vi "Experiment_Disp_ AttTrav.vi"() -> ()   [LabVIEW 2009]
uses:
  <vilib>/imath/engines/lvmath2/RunTimeEngine/ErrorHandling/NIMS_Finalize Error.vi
  <vilib>/imath/engines/lvmath2/RunTimeEngine/Parser/MC_Version.vi
  <vilib>/imath/engines/lvmath/Functions/Error Handling/error.ctl
  <vilib>/imath/engines/lvmath2/RunTimeEngine/RangeToken/NIMS_Range.vi
  <instcachedir>/0/NIMS_Range_6D647EC16A744C98B5DE1D649A2D648D.lvgen/NIMS_Range_6D647EC16A744C98B5DE1D649A2D648D_001.vi
  <vilib>/imath/engines/lvmath/Functions/Error Handling/MergeErrorsWrapper.vi
  <vilib>/imath/engines/lvmath2/RunTimeEngine/VariableToken/NIMS_VariableToken_CondDefined.vi
  <instcachedir>/0/NIMS_VariableToken_CondDefined_5641E79000FB4D628475532441475385.lvgen/NIMS_VariableToken_CondDefined_5641E79000FB4D628475532441475385_002.vi
  <instcachedir>/0/NIMS_VariableToken_CondDefined_5641E79000FB4D628475532441475385.lvgen/NIMS_VariableToken_CondDefined_5641E79000FB4D628475532441475385_001.vi
  <vilib>/imath/engines/lvmath/Functions/Error Handling/MC_Mask_Errors.vi
  <vilib>/imathl/engines/lvmath/Functions/Error Handling/Create Error.vi
  <vilib>/imath/engines/lvmath2/RunTimeEngine/ReplaceToken/NIMS_Replace - V(S)=S.vi
  <instcachedir>/0/NIMS_Replace - V(S)=S_670A9E0533664C1D848C8E58B3321B6A.lvgen/NIMS_Replace - V(S)=S_670A9E0533664C1D848C8E58B3321B6A_000.vi
  <vilib>/imath/engines/lvmath2/RunTimeEngine/ReplaceToken/NIMS_Replace - Size Check _(_)=S.vi
  <instcachedir>/0/NIMS_Replace - Size Check _(_)=S_8596181D73404097BAB9CBB006194BB0.lvgen/NIMS_Replace - Size Check _(_)=S_8596181D73404097BAB9CBB006194BB0_001.vi
  <vilib>/imath/engines/lvmath2/RunTimeEngine/ReplaceToken/NIMS_Replace - Check Linear.vi
  <instcachedir>/0/NIMS_Replace - Check Linear_9243CBB174894FF6977027453DA6955E.lvgen/NIMS_Replace - Check Linear_9243CBB174894FF6977027453DA6955E_001.vi
  <vilib>/imath/engines/lvmath2/RunTimeEngine/VariableToken/NIMS_VariableToken_CondDefinedDefinedByReplace.vi
  <instcachedir>/0/NIMS_VariableToken_CondDefinedDefinedByReplace_D162CFFC24174562A9FEA619A91E1A56.lvgen/NIMS_VariableToken_CondDefinedDefinedByReplace_D162CFFC24174562A9FEA619A91E1A56_001.vi
  <instcachedir>/0/NIMS_Replace - V(S)=S_670A9E0533664C1D848C8E58B3321B6A.lvgen/NIMS_Replace - V(S)=S_670A9E0533664C1D848C8E58B3321B6A_001.vi
  <instcachedir>/0/NIMS_Replace - Size Check _(_)=S_8596181D73404097BAB9CBB006194BB0.lvgen/NIMS_Replace - Size Check _(_)=S_8596181D73404097BAB9CBB006194BB0_002.vi
  <instcachedir>/0/NIMS_Replace - Check Linear_9243CBB174894FF6977027453DA6955E.lvgen/NIMS_Replace - Check Linear_9243CBB174894FF6977027453DA6955E_002.vi
  <instcachedir>/0/NIMS_VariableToken_CondDefinedDefinedByReplace_D162CFFC24174562A9FEA619A91E1A56.lvgen/NIMS_VariableToken_CondDefinedDefinedByReplace_D162CFFC24174562A9FEA619A91E1A56_002.vi
  <vilib>/imath/engines/lvmath2/RunTimeEngine/CommandStatement/MC_CommandStatement_break.vi
  <vilib>/imath/engines/lvmath2/RunTimeEngine/Managers/WorkSpace/UID Generator.vi
  <vilib>/imath/engines/lvmath2/RunTimeEngine/Managers/SymbolTable/Clear UID.vi
  <instcachedir>/0/NIMS_VariableToken_CondDefined_5641E79000FB4D628475532441475385.lvgen/NIMS_VariableToken_CondDefined_5641E79000FB4D628475532441475385_003.vi
  <instcachedir>/0/NIMS_Replace - V(S)=S_670A9E0533664C1D848C8E58B3321B6A.lvgen/NIMS_Replace - V(S)=S_670A9E0533664C1D848C8E58B3321B6A_002.vi
  <instcachedir>/0/NIMS_Replace - Size Check _(_)=S_8596181D73404097BAB9CBB006194BB0.lvgen/NIMS_Replace - Size Check _(_)=S_8596181D73404097BAB9CBB006194BB0_003.vi
  <vilib>/imath/engines/lvmath2/RunTimeEngine/ArithmeticOperatorToken/NIMS_ArithmeticOperator_power(S).vi
  <instcachedir>/0/NIMS_ArithmeticOperator_power(S)_A502679C095F4520BDC53E297C98A9BD.lvgen/NIMS_ArithmeticOperator_power(S)_A502679C095F4520BDC53E297C98A9BD_000.vi
  <instcachedir>/0/NIMS_Replace - Check Linear_9243CBB174894FF6977027453DA6955E.lvgen/NIMS_Replace - Check Linear_9243CBB174894FF6977027453DA6955E_003.vi
  <instcachedir>/0/NIMS_VariableToken_CondDefinedDefinedByReplace_D162CFFC24174562A9FEA619A91E1A56.lvgen/NIMS_VariableToken_CondDefinedDefinedByReplace_D162CFFC24174562A9FEA619A91E1A56_003.vi
  <vilib>/imath/engines/lvmath2/RunTimeEngine/LocalVariableDefStatement/MC_LocalVariableDefStatement_Display.vi
  <vilib>/imath/engines/lvmath2/RunTimeEngine/RunTimeType/NIMS_RunTimeType_From StrictType (excl LVString).vi
  <vilib>/imath/engines/lvmath2/RunTimeEngine/VariableToken/Read/NIMS_Get Elements - RV(_) - Check.vi
  <instcachedir>/0/NIMS_Get Elements - RV(_) - Check_60F12861D0564803969A5D0D0D1716CD.lvgen/NIMS_Get Elements - RV(_) - Check_60F12861D0564803969A5D0D0D1716CD_002.vi
  <vilib>/imath/engines/lvmath2/RunTimeEngine/Managers/SymbolTable/NIMS_WorkSpace.lvlib
panel:
  out "error out":errorcluster
  out "error out":errorcluster
  out "error out":errorcluster
  in  "?":enum32{"TRANSMISSION LINE DEMONSTRATOR"}(tab)
  out "?":cluster{"Y":dbl[], "Y":dbl[]}[](graph)
  in  "Delay Time (s)":dbl min=0.0 step=0.005
  in  "HELP FOR TLD":bool
  in  "?":enum32{"OSCILOSCOPE"}(tab)
  out "?":cluster{"Y":dbl[], "Y":dbl[]}[](graph)
  in  "HELP FOR CRO":bool
  in  "?":enum32{"SOURCE"}(tab)
  out "?":cluster{"Y":dbl[], "Y":dbl[]}[](graph)
  in  "HELP FOR SOURCE":bool
  in  "?":bool
  # "Transmission line demonstrator"
  # "Osciloscope"
  # "Function generator"
  # "ON"
  # "OFF"
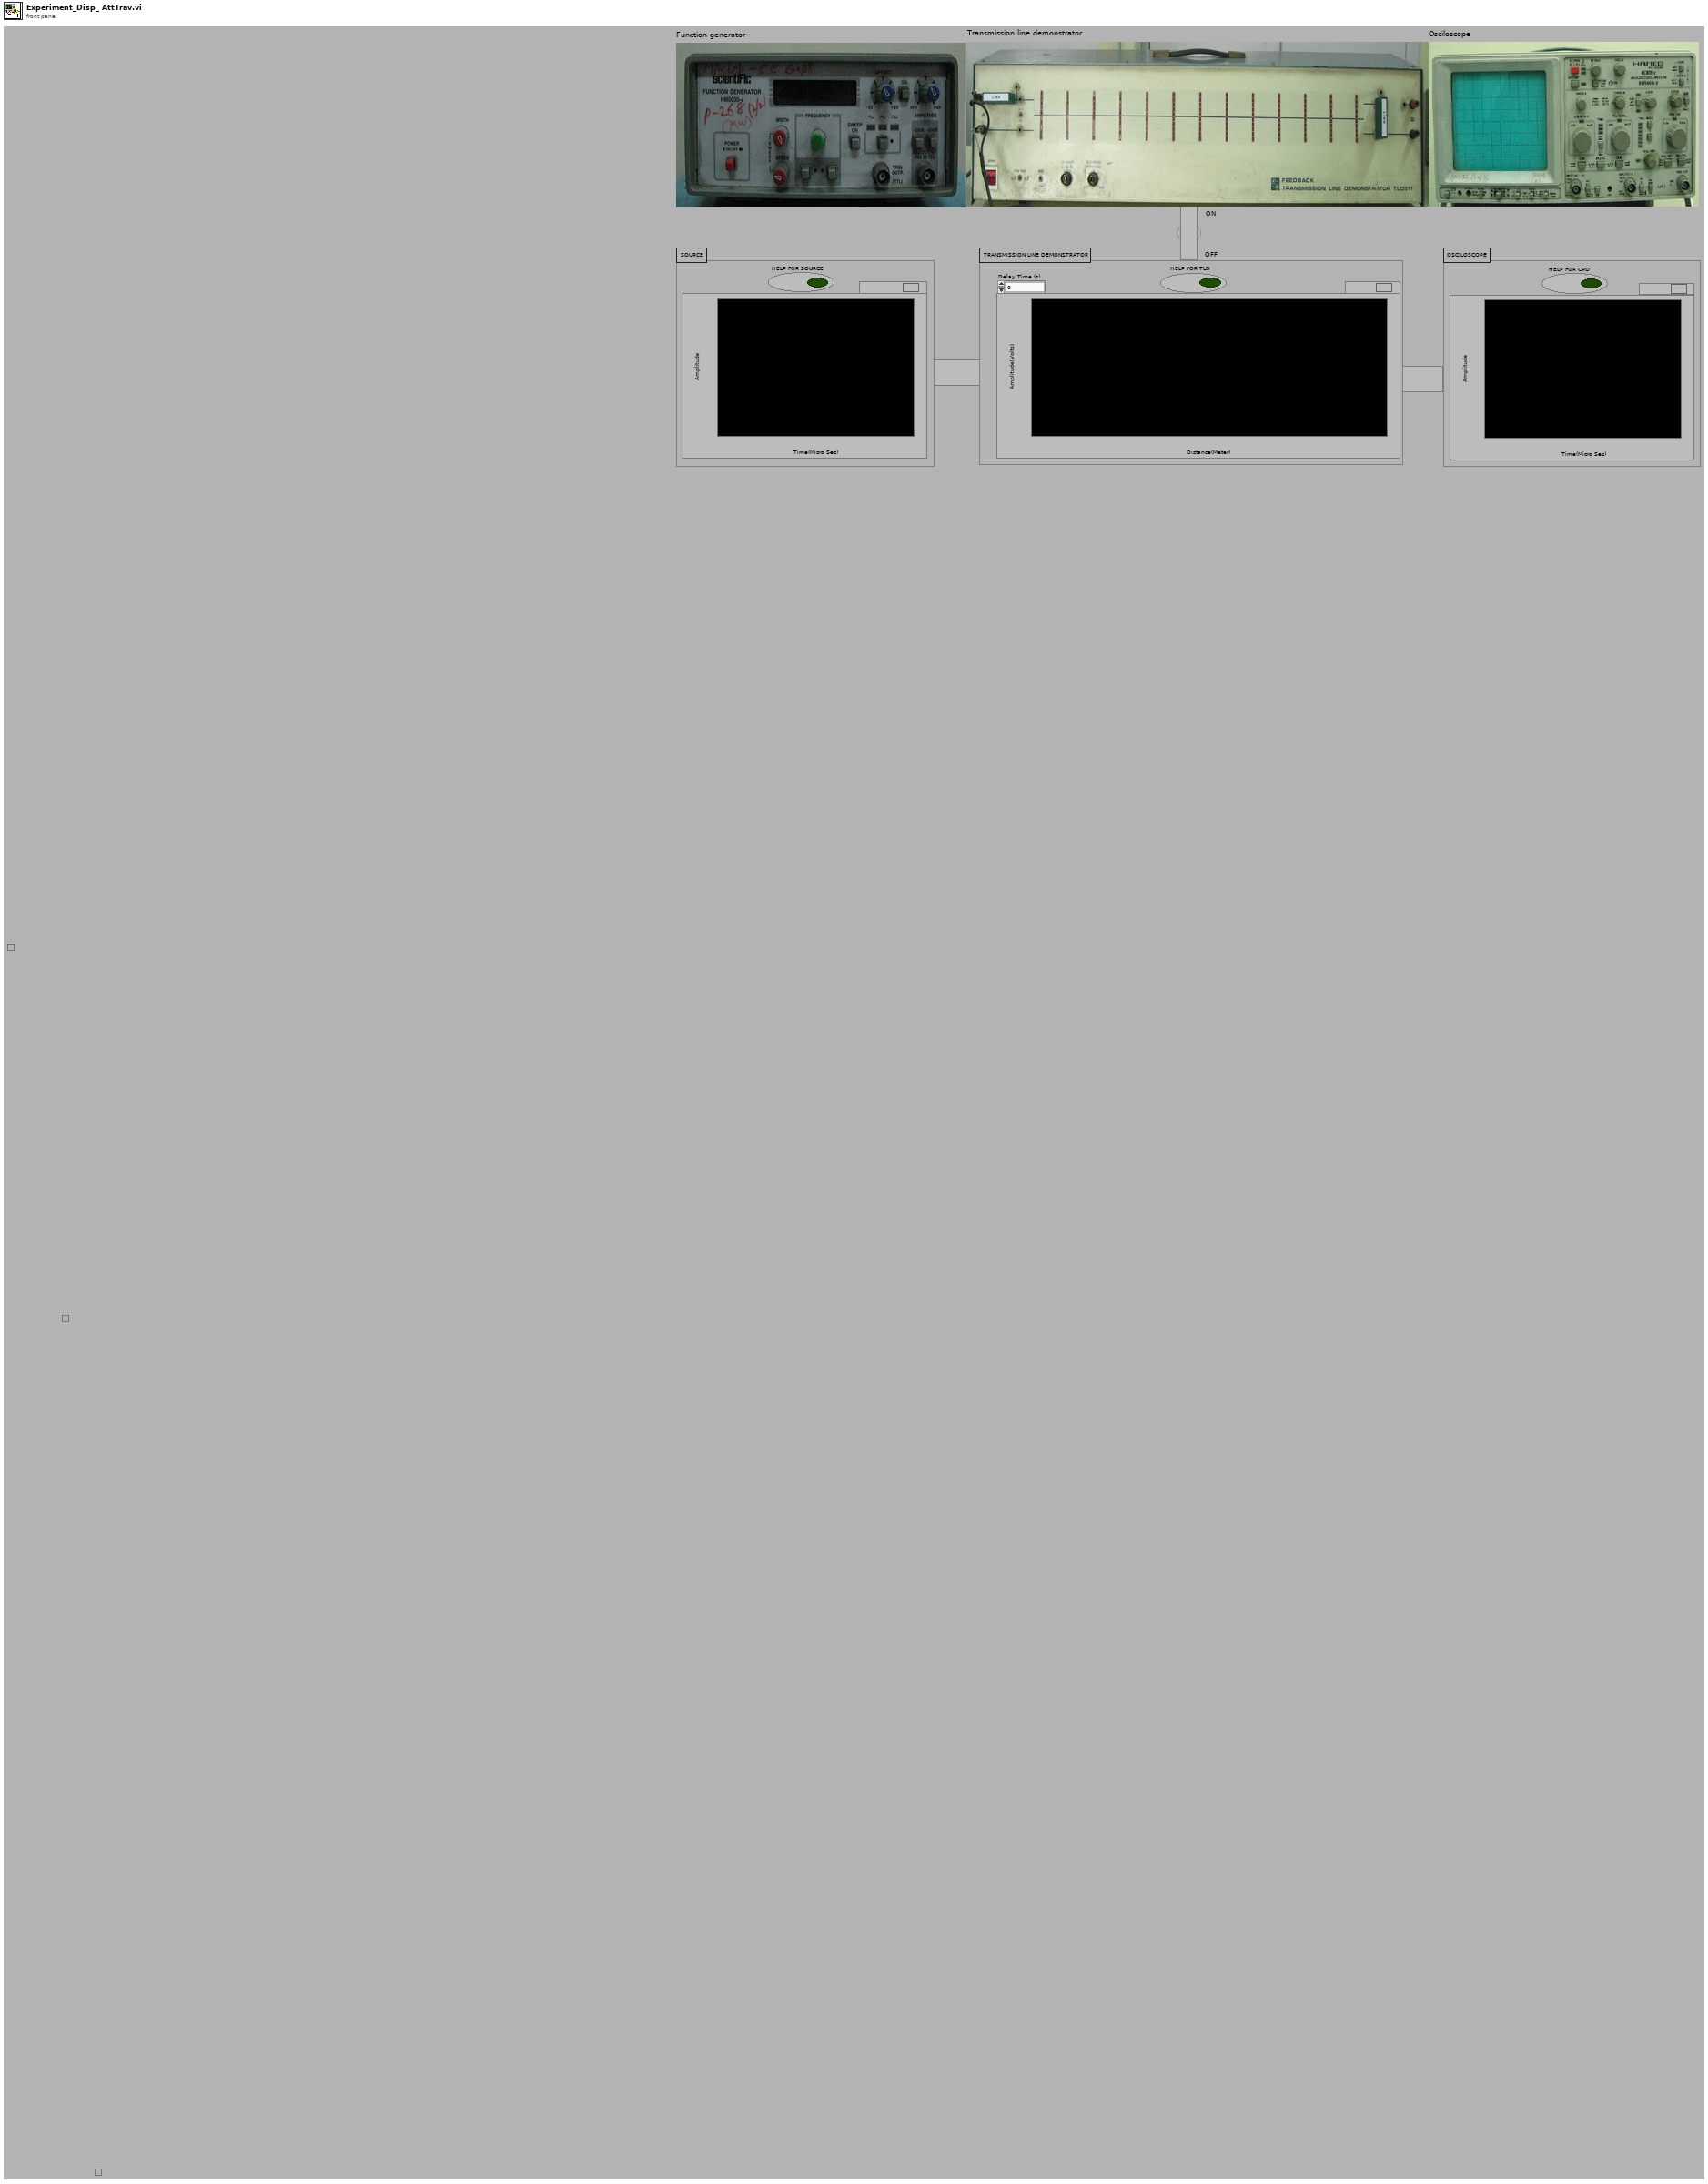
[diagram p1: front panel]
types:
  T1 = typedef "error.ctl" = enum16{"No Error", "Problem", "Unused002", "Incorrect number of parameters", "Function not defined for non-numeric types", "Unused005", "Function only defined for character arrays", "Function not defined for boolean, character, or single precision", "Function not defined for complex types", "Not a valid operation", "Inputs must be scalar", "Input matrices are not the same size", "Unused012", "Input matrices must be nonnegative integers of the same type", "Arguments must be non-negative integers less than bitmax", "Number to complement must be less than 2^N", "Bit to get is outside range", "Bit to set is outside range", "Input must be real type ", "At least one parameter must be scalar", "Unused020", "Function not defined for\nhigher dimensional matrices.", "Invalid attributes", "Wrong Type of Input Arguments", "Wrong Argument Option", "Unused025", "Indices must be real positive integers", "Unused027", "Number of elements must be the same for indices and values", "Unused029", "Cannot resize a 2D matrix with a linear index", "Unknown variable or symbol", "Indices out of range", "Empty matrix deletion can not be used with two indices", "Number of rows and columns must be the same for indices and values.", "Complex cannot be converted to Boolean", "Char cannot be converted to Boolean", "int64 cannot be converted to Boolean", "uint64 cannot be converted to Boolean", "Unused039", "Unused040", "All rows must have the same number of columns", "Incompatible types", "Invalid matrix dimensions", "Dimension must be 1 or 2", "Base must be an integer between 2 and 36", "Invalid input", "Square matrix required", "Function 'timerstart' must be called before 'timerstop'", "Arguments must be positive real", "Step must not be zero", "Wrong number of input arguments", "Wrong number of output arguments", "Unused053", "Input scalar must be >= 0", "Input scalar must be positive", "Input scalar must not be 0", "Input scalar must be in range [0,1]", "Unused058", "Input must be a vector", "Unused060", "Empty vector error", "All elements must be in domain [-1,1]", "All real elements of input vector must be >= 0", "All elements of input vector must be positive", "Values of input vectors are not compatible", "Unused066", "Input vector must be an increasing vector", "Unused068", "Unused069", "Lenths of two input vectors are not compatible", "Unused071", "Empty matrix error", "Unused073", "Unused074", "Unused075", "Unused076", "Unused077", "Size of input matrix is incompatible with input size", "Invalid format specifier", "Unused080", "Unused081", "Unused082", "Unused083", "Unused084", "Unused085", "RunTime: MathScript could not be compiled", "Unknown function", "Only scalars and strings supported", "Unused089", "Unused090", "Range is too large", "End used without variable", "Function not available (RTE)", "Custom user error", "Arguments must be integers less than bitmax", "Shared library not found", "Header file not found", "Shared library already loaded", "Shared library not loaded", "Shared library function not found", "Shared library string return problem", "Problem calling shared library function", "Problem loading shared library from OS", "Problem parsing shared library header file", "Shared library incompatible types", "Shared library unsupported return type", "Shared library function not exported", "Shared library unsupported input type", "Problem unloading shared library from OS", "Function only available from UI", "Invalid function specified in argument", "An internal error has occurred", "Invalid object", "Invalid property", "Read-only property", "A break command has occurred", "A continue command has occurred", "A return command has occurred", "ode: times parameter invalid", "Unused120", "Function not found in file", "Reserved keyword cannot be defined as variable", "Reserved keyword cannot be defined as a function or script", "Arguments must be string literals", "Function not supported on this platform", "All columns must have the same number of rows", "Function ignored in RTE warning", "Cannot use : as a parameter that is not a variable", "Output can't be coerced to requested type", "Function not supported on current target", "Variable dependent on an unwired function input", "Unused132", "Unused133", "Unused134", "Unused135", "Unused136", "Unused137", "Unused138", "Unused139", "Unused140", "Unused141", "Unused142", "Unused143", "Unused144", "Unused145", "Unused146", "MathScript parser DLL missing", "MathScript requires LabVIEW Full", "MathScript license is invalid or missing"}
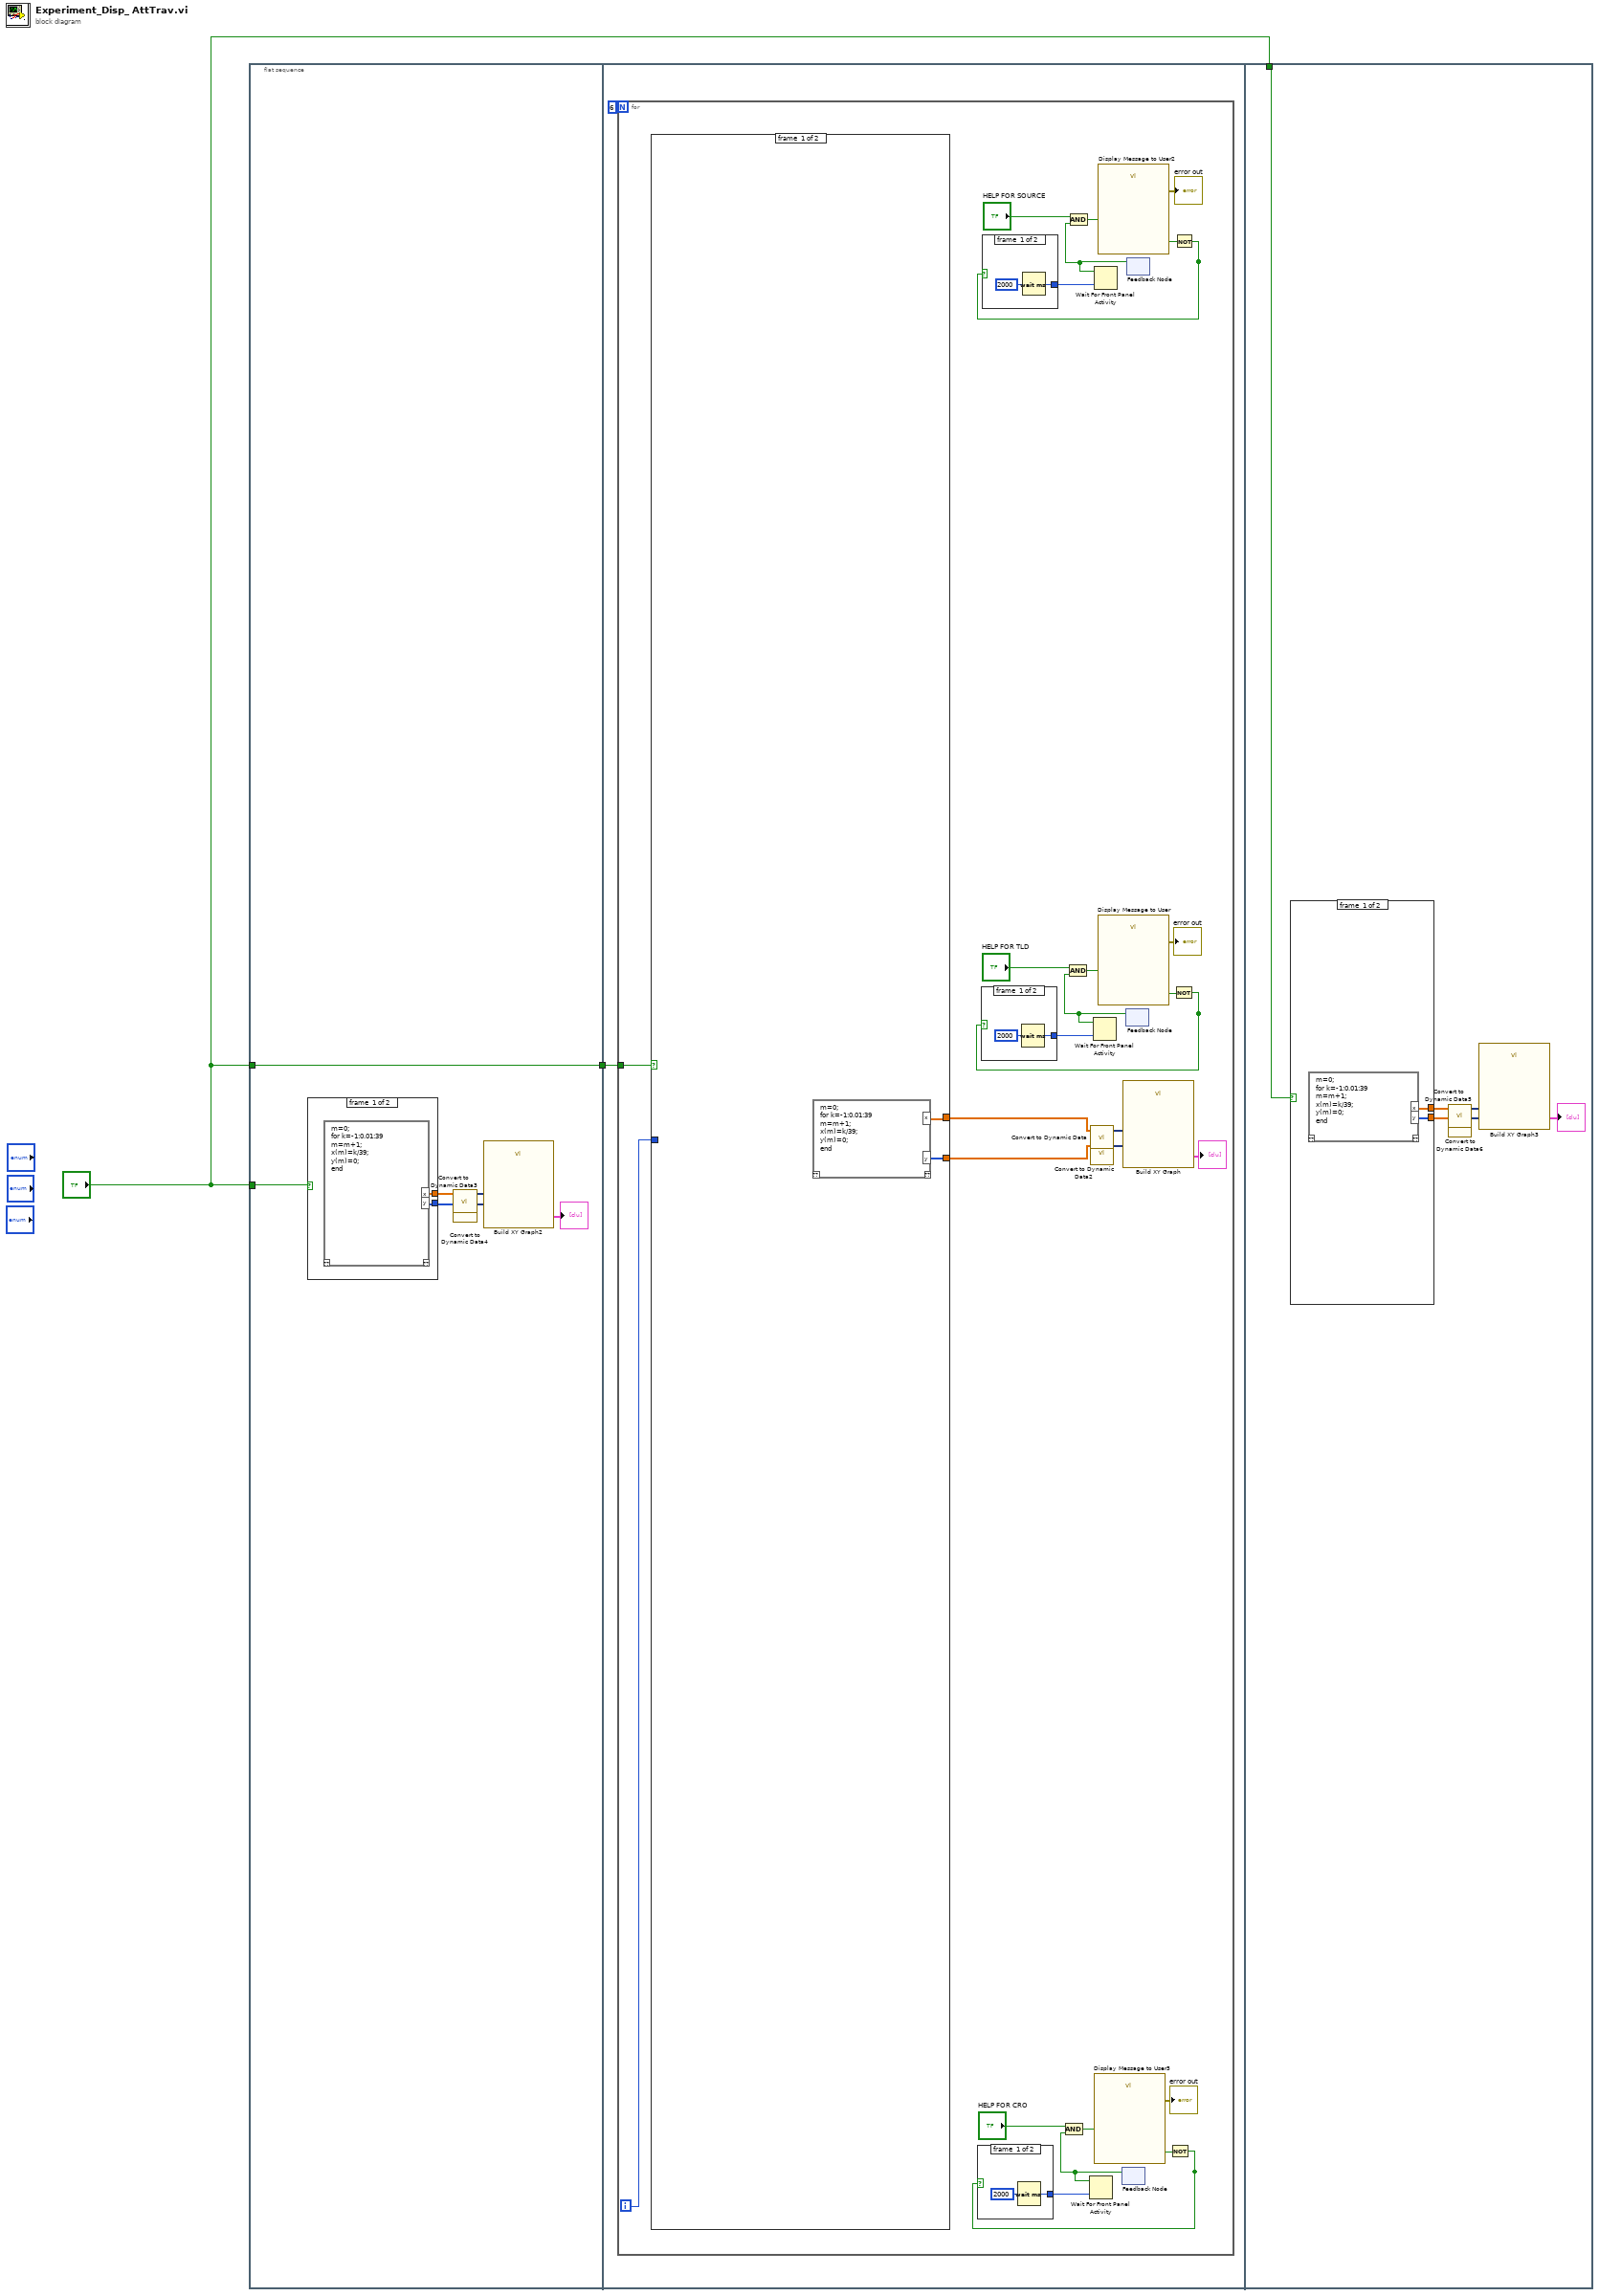
[diagram p0: block diagram]
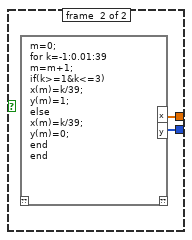
[diagram p2: hidden frame]
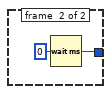
[diagram p3: hidden frame]
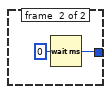
[diagram p4: hidden frame]
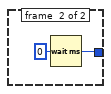
[diagram p5: hidden frame]
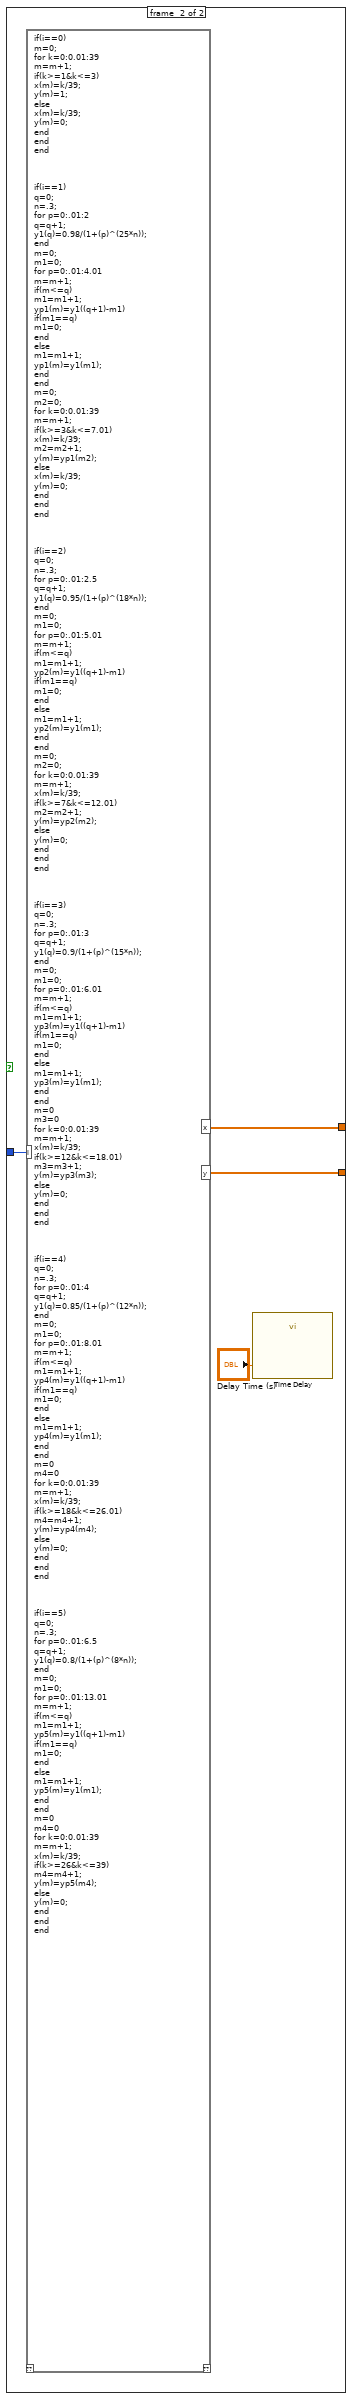
[diagram p6: hidden frame]
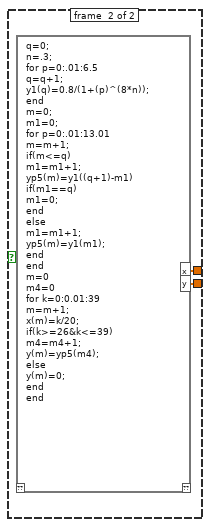
[diagram p7: hidden frame]
diagram:
  n1 = flat-sequence {
    tunnel: [w4] -> w2
    tunnel: "?" -> [w4]
    tunnel: "?" -> [w3]
    tunnel: w2 -> [w338]
    tunnel: "?" -> [w3370]
    frame #0 {
      n2 = case shown="True" w3 {
        tunnel: [w10 w146] -> w9
        tunnel: [w11 w145] -> w7
        frame #0 {
          n3 = mathscript code="m=0;\nfor k=-1:0.01:39\nm=m+1;\nx(m)=k/39;\ny(m)=0;\nend"() -> ("x"=w10:dbl[], "y"=w11:i32[])  [unwired: 1 in, 1 out]
        }
        frame #1 {
          n4 = mathscript code="m=0;\nfor k=-1:0.01:39\nm=m+1;\nif(k>=1&k<=3)\nx(m)=k/39;\ny(m)=1;\nelse\nx(m)=k/39;\ny(m)=0;\nend\nend"() -> ("x"=w146:dbl[], "y"=w145:i32[])  [unwired: 1 in, 1 out]
        }
      }
      n5 = call "Convert to Dynamic Data3"("Array"=w9) -> ("Dynamic Data Type"=w8:dynamicdata)  [unwired: 3 in]
      n6 = call "Convert to Dynamic Data4"("Array"=w7) -> ("Dynamic Data Type"=w6:dynamicdata)  [unwired: 3 in]
      n7 = call "Build XY Graph2"("Y Input"=w6, "X Input"=w8) -> ("XY Graph"=→"?":cluster{"Y":dbl[], "Y":dbl[]}[])  [unwired: 8 in, 1 out]
    }
    frame #1 {
      n8 = for {
        N: 6 -> [_]
        tunnel: w338 -> [w361]
        i -> [w367]
        n9 = case shown="True" w361 {
          tunnel: w367 -> [_ w518]
          tunnel: [w381 w517] -> w363
          tunnel: [w380 w516] -> w362
          frame #0 {
            n10 = mathscript code="m=0;\nfor k=-1:0.01:39\nm=m+1;\nx(m)=k/39;\ny(m)=0;\nend"() -> ("x"=w381:dbl[], "y"=w380:i32[])  [unwired: 1 in, 1 out]
          }
          frame #1 {
            n11 = mathscript code="if(i==0)\nm=0;\nfor k=0:0.01:39\nm=m+1;\nif(k>=1&k<=3)\nx(m)=k/39;\ny(m)=1;\nelse\nx(m)=k/39;\ny(m)=0;\nend\nend\nend\n\n\n\nif(i==1)\nq=0;\nn=.3;\nfor p=0:.01:2\nq=q+1;\ny1(q)=0.98/(1+(p)^(25*n));\nend\nm=0;\nm1=0;\nfor p=0:.01:4.01\nm=m+1;\nif(m<=q)\nm1=m1+1;\nyp1(m)=y1((q+1)-m1)\nif(m1==q)\nm1=0;\nend\nelse\nm1=m1+1;\nyp1(m)=y1(m1);\nend\nend\nm=0;\nm2=0;\nfor k=0:0.01:39\nm=m+1;\nif(k>=3&k<=7.01)\nx(m)=k/39;\nm2=m2+1;\ny(m)=yp1(m2);\nelse\nx(m)=k/39;\ny(m)=0;\nend\nend\nend\n\n\n\nif(i==2)\nq=0;\nn=.3;\nfor p=0:.01:2.5\nq=q+1;\ny1(q)=0.95/(1+(p)^(18*n));\nend\nm=0;\nm1=0;\nfor p=0:.01:5.01\nm=m+1;\nif(m<=q)\nm1=m1+1;\nyp2(m)=y1((q+1)-m1)\nif(m1==q)\nm1=0;\nend\nelse\nm1=m1+1;\nyp2(m)=y1(m1);\nend\nend\nm=0;\nm2=0;\nfor k=0:0.01:39\nm=m+1;\nx(m)=k/39;\nif(k>=7&k<=12.01)\nm2=m2+1;\ny(m)=yp2(m2);\nelse\ny(m)=0;\nend\nend\nend\n\n\n\nif(i==3)\nq=0;\nn=.3;\nfor p=0:.01:3\nq=q+1;\ny1(q)=0.9/(1+(p)^(15*n));\nend\nm=0;\nm1=0;\nfor p=0:.01:6.01\nm=m+1;\nif(m<=q)\nm1=m1+1;\nyp3(m)=y1((q+1)-m1)\nif(m1==q)\nm1=0;\nend\nelse\nm1=m1+1;\nyp3(m)=y1(m1);\nend\nend\nm=0\nm3=0\nfor k=0:0.01:39\nm=m+1;\nx(m)=k/39;\nif(k>=12&k<=18.01)\nm3=m3+1;\ny(m)=yp3(m3);\nelse\ny(m)=0;\nend\nend\nend\n\n\n\nif(i==4)\nq=0;\nn=.3;\nfor p=0:.01:4\nq=q+1;\ny1(q)=0.85/(1+(p)^(12*n));\nend\nm=0;\nm1=0;\nfor p=0:.01:8.01\nm=m+1;\nif(m<=q)\nm1=m1+1;\nyp4(m)=y1((q+1)-m1)\nif(m1==q)\nm1=0;\nend\nelse\nm1=m1+1;\nyp4(m)=y1(m1);\nend\nend\nm=0\nm4=0\nfor k=0:0.01:39\nm=m+1;\nx(m)=k/39;\nif(k>=18&k<=26.01)\nm4=m4+1;\ny(m)=yp4(m4);\nelse\ny(m)=0;\nend\nend\nend\n\n\n\nif(i==5)\nq=0;\nn=.3;\nfor p=0:.01:6.5\nq=q+1;\ny1(q)=0.8/(1+(p)^(8*n));\nend\nm=0;\nm1=0;\nfor p=0:.01:13.01\nm=m+1;\nif(m<=q)\nm1=m1+1;\nyp5(m)=y1((q+1)-m1)\nif(m1==q)\nm1=0;\nend\nelse\nm1=m1+1;\nyp5(m)=y1(m1);\nend\nend\nm=0\nm4=0\nfor k=0:0.01:39\nm=m+1;\nx(m)=k/39;\nif(k>=26&k<=39)\nm4=m4+1;\ny(m)=yp5(m4);\nelse\ny(m)=0;\nend\nend\nend"("i"=w518) -> ("x"=w517:dbl[], "y"=w516:cdb[])  [unwired: 1 in, 1 out]
            n12 = call "Time Delay"("Delay Time (s)"="Delay Time (s)") -> ()  [unwired: 10 in, 1 out]
          }
        }
        n13 = call "Convert to Dynamic Data"("Array"=w363) -> ("Dynamic Data Type"=w365:dynamicdata)  [unwired: 3 in]
        n14 = call "Convert to Dynamic Data2"("Array"=w362) -> ("Dynamic Data Type"=w364:dynamicdata)  [unwired: 3 in]
        n15 = feedback #1() -> (w344:bool)  [unwired: 1 in]
        n16 = And(x="HELP FOR CRO", y=w344) -> (x .and. y?=w345:bool)
        n17 = call "Display Message to User3"("Enable"=w345) -> ("error out"=→"error out":errorcluster, "CLOSE"=w343:bool)  [unwired: 2 in, 7 out]
        n18 = call "Build XY Graph"("Y Input"=w364, "X Input"=w365) -> ("XY Graph"=→"?":cluster{"Y":dbl[], "Y":dbl[]}[])  [unwired: 3 in, 6 out]
        n19 = feedback #2() -> (w351:bool)  [unwired: 1 in]
        n20 = And(x="HELP FOR TLD", y=w351) -> (x .and. y?=w352:bool)
        n21 = call "Display Message to User"("Enable"=w352) -> ("error out"=→"error out":errorcluster, "CLOSE"=w350:bool)  [unwired: 2 in, 7 out]
        n22 = feedback #3() -> (w358:bool)  [unwired: 1 in]
        n23 = And(x="HELP FOR SOURCE", y=w358) -> (x .and. y?=w359:bool)
        n24 = call "Display Message to User2"("Enable"=w359) -> ("error out"=→"error out":errorcluster, "CLOSE"=w357:bool)  [unwired: 2 in, 7 out]
        n25 = Not(x=w343) -> (.not. x?=w341:bool)
        n26 = case shown="False" w341 {
          tunnel: [w368 w370] -> w340
          frame #0 {
            n27 = Wait (ms)(milliseconds to wait=u32 2000) -> (millisecond timer value=w368:u32)
          }
          frame #1 {
            n28 = Wait (ms)(milliseconds to wait=u32 0) -> (millisecond timer value=w370:u32)
          }
        }
        n29 = Wait For Front Panel Activity(1:w340, 3:w344) -> ()  [unwired: 1 in, 1 out]
        n30 = Not(x=w350) -> (.not. x?=w348:bool)
        n31 = case shown="False" w348 {
          tunnel: [w372 w374] -> w347
          frame #0 {
            n32 = Wait (ms)(milliseconds to wait=u32 2000) -> (millisecond timer value=w372:u32)
          }
          frame #1 {
            n33 = Wait (ms)(milliseconds to wait=u32 0) -> (millisecond timer value=w374:u32)
          }
        }
        n34 = Wait For Front Panel Activity(1:w347, 3:w351) -> ()  [unwired: 1 in, 1 out]
        n35 = Not(x=w357) -> (.not. x?=w355:bool)
        n36 = case shown="False" w355 {
          tunnel: [w376 w378] -> w354
          frame #0 {
            n37 = Wait (ms)(milliseconds to wait=u32 2000) -> (millisecond timer value=w376:u32)
          }
          frame #1 {
            n38 = Wait (ms)(milliseconds to wait=u32 0) -> (millisecond timer value=w378:u32)
          }
        }
        n39 = Wait For Front Panel Activity(1:w354, 3:w358) -> ()  [unwired: 1 in, 1 out]
      }
    }
    frame #2 {
      n40 = case shown="True" w3370 {
        tunnel: [w3377 w3512] -> w3375
        tunnel: [w3376 w3511] -> w3371
        frame #0 {
          n41 = mathscript code="m=0;\nfor k=-1:0.01:39\nm=m+1;\nx(m)=k/39;\ny(m)=0;\nend"() -> ("x"=w3377:dbl[], "y"=w3376:i32[])  [unwired: 1 in, 1 out]
        }
        frame #1 {
          n42 = mathscript code="q=0;\nn=.3;\nfor p=0:.01:6.5\nq=q+1;\ny1(q)=0.8/(1+(p)^(8*n));\nend\nm=0;\nm1=0;\nfor p=0:.01:13.01\nm=m+1;\nif(m<=q)\nm1=m1+1;\nyp5(m)=y1((q+1)-m1)\nif(m1==q)\nm1=0;\nend\nelse\nm1=m1+1;\nyp5(m)=y1(m1);\nend\nend\nm=0\nm4=0\nfor k=0:0.01:39\nm=m+1;\nx(m)=k/20;\nif(k>=26&k<=39)\nm4=m4+1;\ny(m)=yp5(m4);\nelse\ny(m)=0;\nend\nend"() -> ("x"=w3512:dbl[], "y"=w3511:cdb[])  [unwired: 1 in, 1 out]
        }
      }
      n43 = call "Convert to Dynamic Data5"("Array"=w3375) -> ("Dynamic Data Type"=w3374:dynamicdata)  [unwired: 3 in]
      n44 = call "Convert to Dynamic Data6"("Array"=w3371) -> ("Dynamic Data Type"=w3373:dynamicdata)  [unwired: 3 in]
      n45 = call "Build XY Graph3"("Y Input"=w3373, "X Input"=w3374) -> ("XY Graph"=→"?":cluster{"Y":dbl[], "Y":dbl[]}[])  [unwired: 8 in, 1 out]
    }
  }
